vi "UDT_admittanceLibrary_Timer FGV.vi"() -> (3 "Unit Test Framework Results":T1)   [LabVIEW 2017]
doc: "Use this template to create a user-defined test VI. Define your test requirements and wire the results to the <b>Result (Test)</b> control. Do not modify the <b>Unit Test Framework Results</b> indicator."
uses:
  <vilib>/utf/common/utf_test_result_troll.ctl
  <vilib>/utf/common/utf_test_result.ctl
  <vilib>/utf/common/utf_test_result_failure.ctl
  <vilib>/utf/common/utf_test_comparison_operators.ctl
  <vilib>/utf/common/utf_vi_tag.ctl
  RT/Admittance Controller/Controls/timer control.ctl
  <vilib>/Control Software Solutions Ltd/UTF Helper/SubVIs/UTF Double Not Equals.vi
  <vilib>/Control Software Solutions Ltd/UTF Helper/SubVIs/UTF Double Equals.vi
  RT/Admittance Controller/admittanceControllerLibrary.lvlib
  <vilib>/Control Software Solutions Ltd/UTF Helper/Unit Test Helper.lvlib
  <vilib>/utf/NI_UnitTestFramework.lvlib
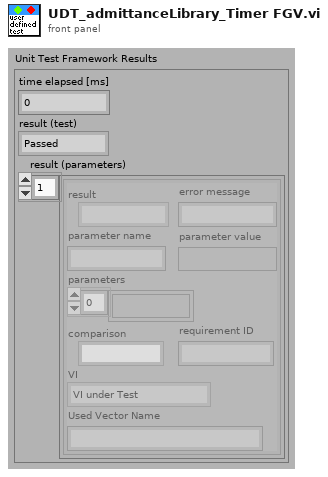
[diagram p1: front panel]
types:
  T1 = typedef "NI_UnitTestFramework.lvlib/utf_test_result_troll.ctl" = cluster{"time elapsed [ms]":u32, "result (test)":T2, "result (parameters)":T3[]}
  T2 = typedef "NI_UnitTestFramework.lvlib/utf_test_result.ctl" = enum16{"Passed", "Failed", "Error", "Skipped", "Not Processed"}
  T3 = typedef "NI_UnitTestFramework.lvlib/utf_test_result_failure.ctl" = cluster{"result":T2, "error message":string, "parameter name":string, "parameter value":variant, "parameters":variant[], "comparison":T4, "requirement ID":string, "VI":T5, "Used Vector Name":string}
  T4 = typedef "NI_UnitTestFramework.lvlib/utf_test_comparison_operators.ctl" = enum16{"=", "!=", ">", ">=", "<", "<=", "range", "symmetric tolerance", "asymmetric tolerance", "string contains", "string not contain", "array size", "string length", "array range", "by element", "array range (limit array)", "user-defined", "array contains", "array not contain", "vector length", "= (elm)", "!= (elm)", "= (case insensitive)", "!= (case insensitive)"}
  T5 = typedef "NI_UnitTestFramework.lvlib/utf_vi_tag.ctl" = enum16{"Setup VI", "VI under Test", "Teardown VI"}
  T6 = typedef "admittanceControllerLibrary.lvlib/timer control.ctl" = enum16{"get time", "set time"}
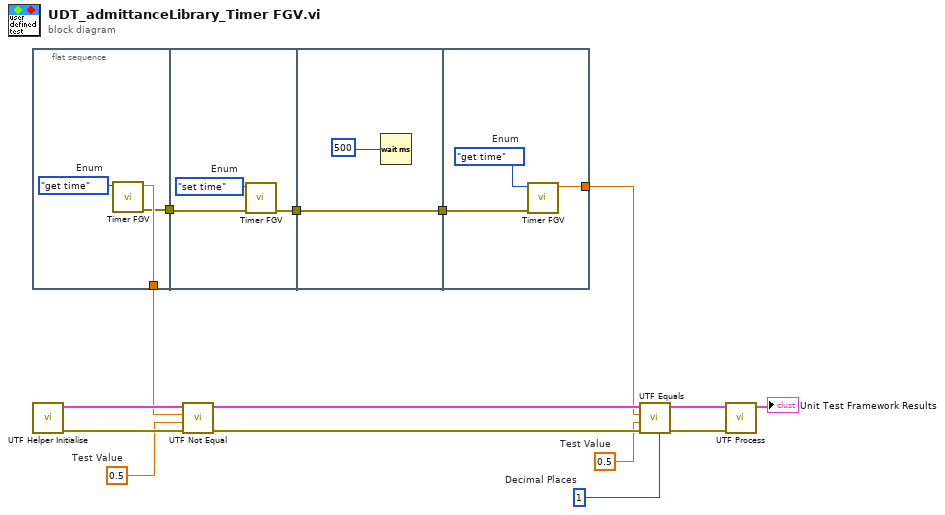
[diagram p0: block diagram]
diagram:
  w1 = u8 1  # Decimal Places
  w3 = 0.5  # Test Value
  w2 = 0.5  # Test Value
  n1 = flat-sequence {
    tunnel: [w17] -> w9
    tunnel: [w16] -> w15
    tunnel: w15 -> [w21]
    tunnel: [w19] -> w14
    tunnel: w14 -> [w23]
    tunnel: [w23] -> w13
    tunnel: w13 -> [w25]
    tunnel: [w24] -> w4
    frame #0 {
      w18 = timer_control."get time"  # Enum
      n2 = call "Timer FGV.vi"("Enum"=w18) -> ("error out"=w16:errorcluster, "Elapsed Time"=w17:dbl)  [unwired: 9 in]
    }
    frame #1 {
      w20 = timer_control."set time"  # Enum
      n3 = call "Timer FGV.vi"("error in (no error)"=w21, "Enum"=w20) -> ("error out"=w19:errorcluster)  [unwired: 8 in, 1 out]
    }
    frame #2 {
      n4 = Wait (ms)(milliseconds to wait=u32 500) -> ()  [unwired: 1 out]
    }
    frame #3 {
      w26 = timer_control."get time"  # Enum
      n5 = call "Timer FGV.vi"("error in (no error)"=w25, "Enum"=w26) -> ("Elapsed Time"=w24:dbl)  [unwired: 8 in, 1 out]
    }
  }
  n6 = call <vilib>:"UTF Helper Initialise.vi"() -> ("error out"=w10:errorcluster, "results array"=w11:T3[])  [unwired: 10 in]
  n7 = call-poly <vilib>:"UTF Not Equal.vi"("error in (no error)"=w10, "Test Value"=w2, "Input"=w9, "Input Results"=w11) -> ("error out"=w5:errorcluster, "Output Results"=w6:T3[])  [unwired: 6 in]
  n8 = call-poly <vilib>:"UTF Equals.vi"("Decimal Places"=w1, "error in (no error)"=w5, "Test Value"=w3, "Input"=w4, "Input Results"=w6) -> ("error out"=w7:errorcluster, "Output Results"=w8:T3[])  [unwired: 5 in]
  n9 = call <vilib>:"UTF Process.vi"("error in (no error)"=w7, "results array"=w8) -> ("Unit Test Framework Results"=→"Unit Test Framework Results":T1)  [unwired: 9 in]
